vi "Manuele override - test.vi"() -> ()   [LabVIEW 2019]
panel:
  out "richtingsaanwijzer":dbl(knob) scale=0.0..10.0
  in  "kruispunt":string
  out "bericht":string
  in  "STOP":bool
  in  "START":bool
  in  "stop 2":bool
  out "address":u32
  out "port":u16
  in  "stop":bool
  in  "vooruit":bool
  in  "achteruit":bool
  in  "links":bool
  in  "rechts":bool
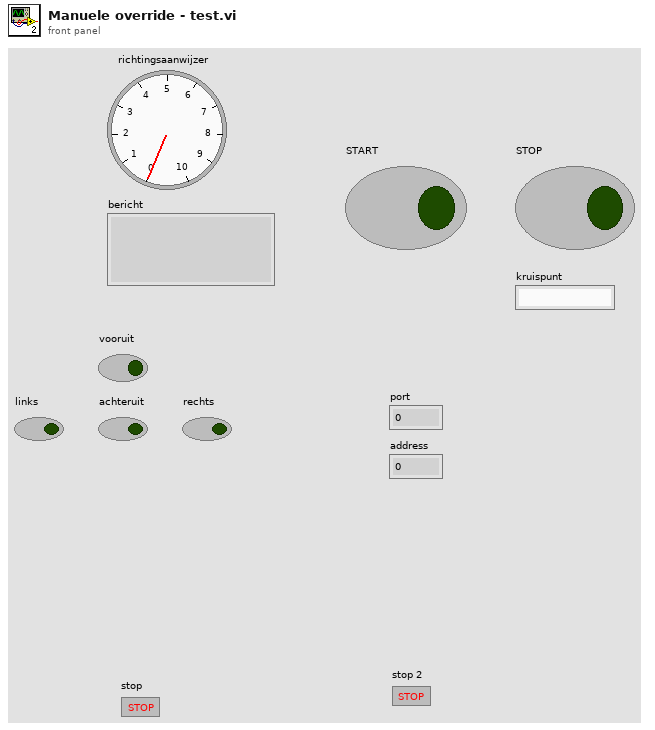
[diagram p1: front panel]
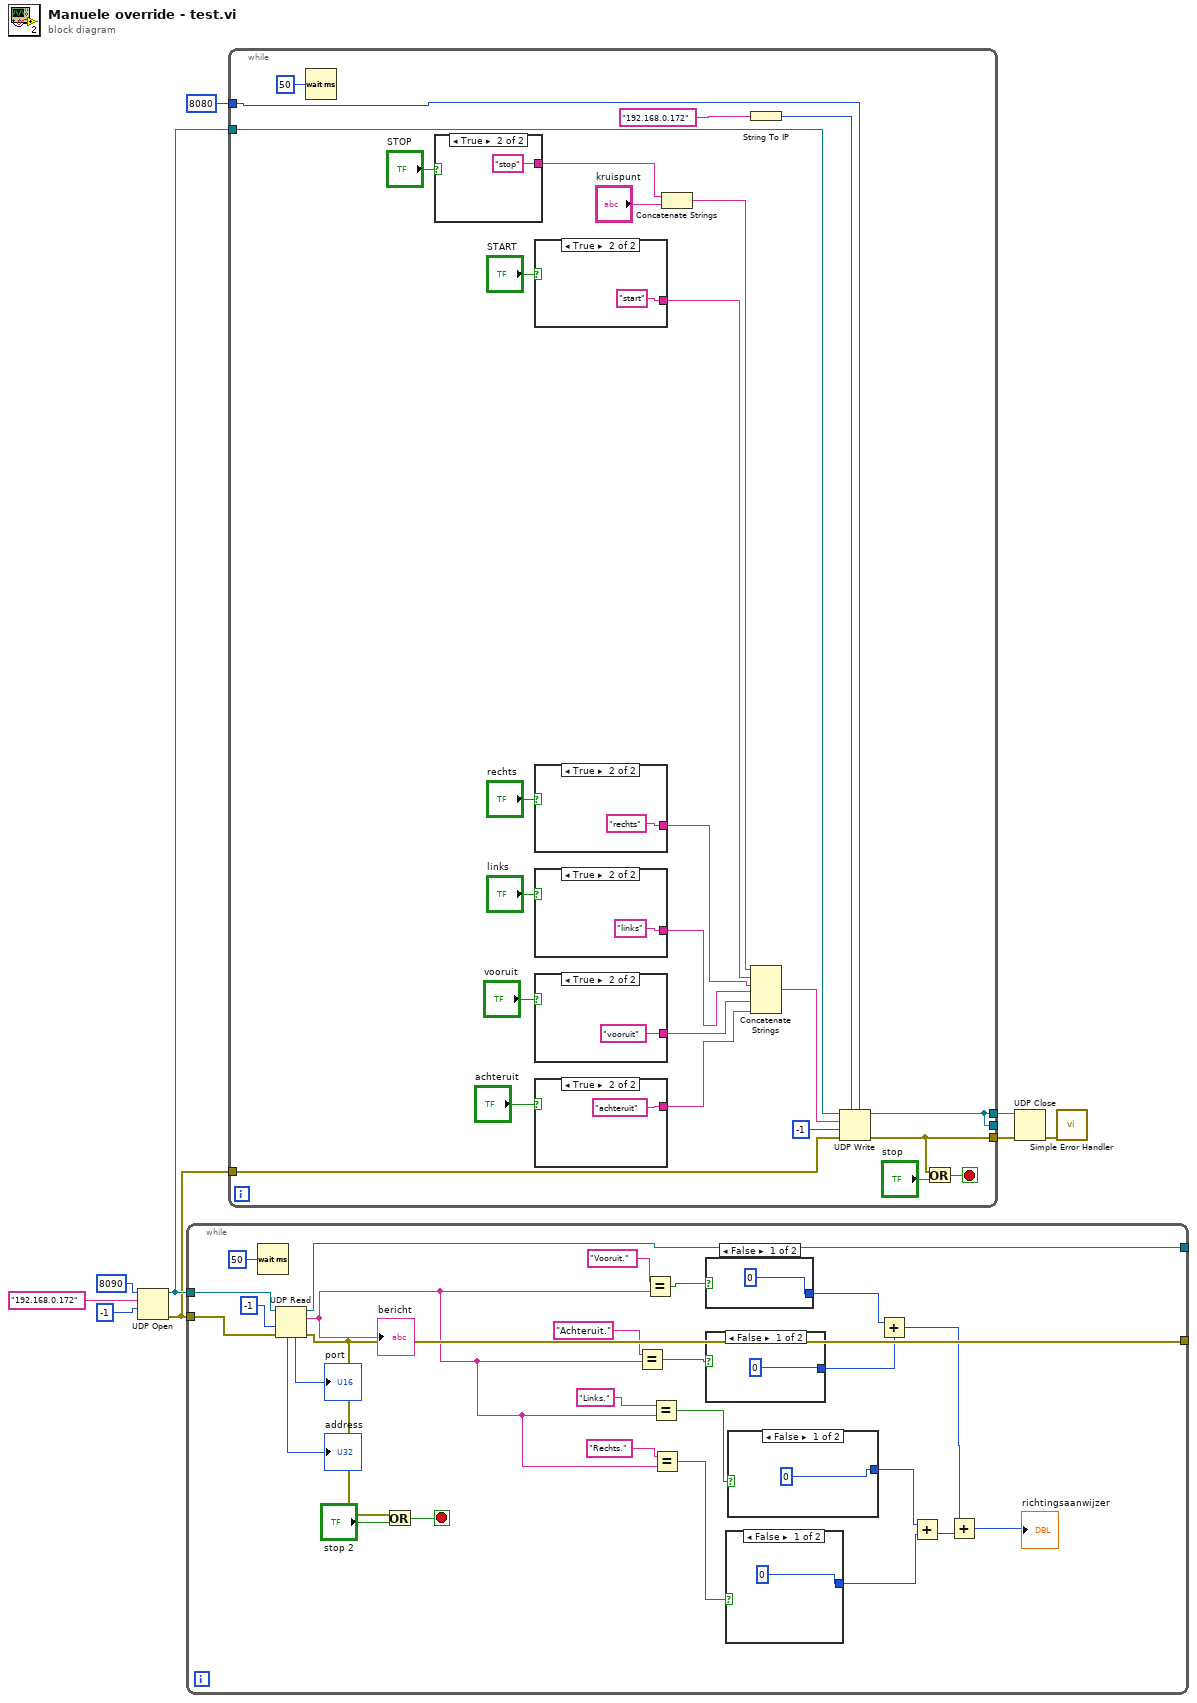
[diagram p0: block diagram]
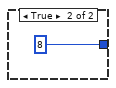
[diagram p2: hidden frame]
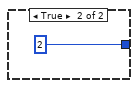
[diagram p3: hidden frame]
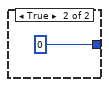
[diagram p4: hidden frame]
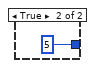
[diagram p5: hidden frame]
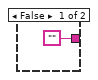
[diagram p6: hidden frame]
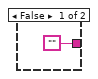
[diagram p7: hidden frame]
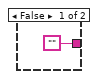
[diagram p8: hidden frame]
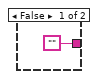
[diagram p9: hidden frame]
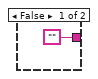
[diagram p10: hidden frame]
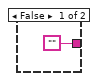
[diagram p11: hidden frame]
diagram:
  n1 = UDP Open(9:-1, 10:"192.168.0.172", 11:8090) -> (port=w5:refnum<k16>, 0:w4:errorcluster)  [unwired: 2 in, 1 out]
  n2 = while {
    tunnel: w5 -> [w35]
    tunnel: w4 -> [w34]
    tunnel: [w31] -> _
    tunnel: [w30] -> _
    stop <- w28 stop-if-true
    n3 = Wait (ms)(milliseconds to wait=u32 50) -> ()  [unwired: 1 out]
    n4 = UDP Read(connection ID=w35, timeout ms (25000)=-1, 8:w34) -> (data out=w20:string, error out=w30:errorcluster, 3:w31:refnum<k16>, 4:→"port":u16, 6:→"address":u32)  [unwired: 1 in]
    "bericht" <- w20
    n5 = Or(x=w30, y="stop 2") -> (x .or. y?=w28:bool)
    n6 = Equal?(x="Achteruit.", y=w20) -> (x = y?=w19:bool)
    n7 = Equal?(x="Vooruit.", y=w20) -> (x = y?=w25:bool)
    n8 = Equal?(x="Links.", y=w20) -> (x = y?=w18:bool)
    n9 = Equal?(x="Rechts.", y=w20) -> (x = y?=w17:bool)
    n10 = case shown="False" w25 {
      tunnel: [0 5] -> w15
      frame False {
      }
      frame True {
      }
    }
    n11 = case shown="False" w19 {
      tunnel: [0 0] -> w16
      frame False {
      }
      frame True {
      }
    }
    n12 = case shown="False" w17 {
      tunnel: [0 8] -> w13
      frame False {
      }
      frame True {
      }
    }
    n13 = case shown="False" w18 {
      tunnel: [0 2] -> w14
      frame False {
      }
      frame True {
      }
    }
    n14 = Add(x=w15, y=w16) -> (x+y=w12:i32)
    n15 = Add(x=w14, y=w13) -> (x+y=w11:i32)
    n16 = Add(x=w12, y=w11) -> (x+y=→"richtingsaanwijzer":i32)
  }
  n17 = while {
    tunnel: w5 -> [w69]
    tunnel: w4 -> [w68]
    tunnel: 8080 -> [w64]
    tunnel: [w55] -> w3
    tunnel: [w63] -> w7
    tunnel: [w55] -> _
    stop <- w66 stop-if-true
    n18 = Wait (ms)(milliseconds to wait=50) -> ()  [unwired: 1 out]
    n19 = case shown="True" "STOP" {
      tunnel: ["" "stop"] -> w50
      frame False {
      }
      frame True {
      }
    }
    n20 = case shown="True" "START" {
      tunnel: ["" "start"] -> w54
      frame False {
      }
      frame True {
      }
    }
    n21 = case shown="True" "rechts" {
      tunnel: ["" "rechts"] -> w47
      frame False {
      }
      frame True {
      }
    }
    n22 = case shown="True" "links" {
      tunnel: ["" "links"] -> w46
      frame False {
      }
      frame True {
      }
    }
    n23 = case shown="True" "vooruit" {
      tunnel: ["" "vooruit"] -> w45
      frame False {
      }
      frame True {
      }
    }
    n24 = case shown="True" "achteruit" {
      tunnel: ["" "achteruit"] -> w44
      frame False {
      }
      frame True {
      }
    }
    n25 = Concatenate Strings(w50, "kruispunt") -> (w51:string)
    n26 = String To IP(1:"192.168.0.172") -> (0:w58:u32)
    n27 = Concatenate Strings(w51, w54, w47, w46, w45, w44) -> (w60:string)
    n28 = UDP Write(address=w58, port or service name=w64, connection ID=w69, data in=w60, 8:w68, 9:-1) -> (error out=w63:errorcluster, 3:w55:refnum<k16>)
    n29 = Or(x=w63, y="stop") -> (x .or. y?=w66:bool)
  }
  n30 = UDP Close(connection ID=w3, 8:w7) -> (error out=w6:errorcluster)  [unwired: 1 out]
  n31 = call <vilib>:"Simple Error Handler.vi"("error in (no error)"=w6) -> ()  [unwired: 4 in, 5 out]
